vi "DynamicLoadLRvi.vi"(0 "LibName\\viName":string="CRC与诊断.lvlibp\\CRC与诊断\\CRC类\\CRC计算.vi", 1 "校验算法名称":string="Anti_Add", 2 "校验数据":u8[](array[numeric])=[215, 130, 0, 0, 0, 0, 11, 0] format="%x", 3 "校验长度":u8=7) -> (14 "校验值":u64=7)   [LabVIEW 2020]
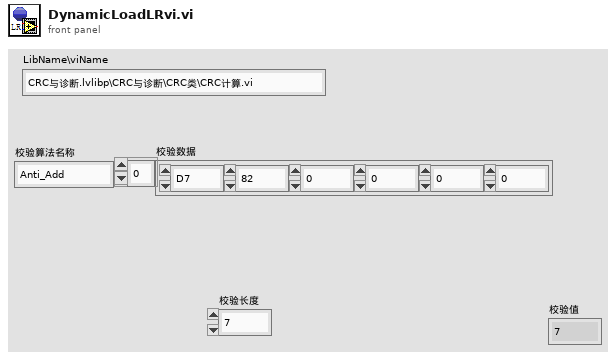
[diagram p1: front panel]
types:
  T1 = enum32{"invalid app kind", "Development System", "Run Time System", "Student Edition", "Embedded LabVIEW", "Evaluation", "Custom"}
  T2 = enum32{"Invalid", "Standard", "Closed", "Hidden", "Minimized", "Maximized"}
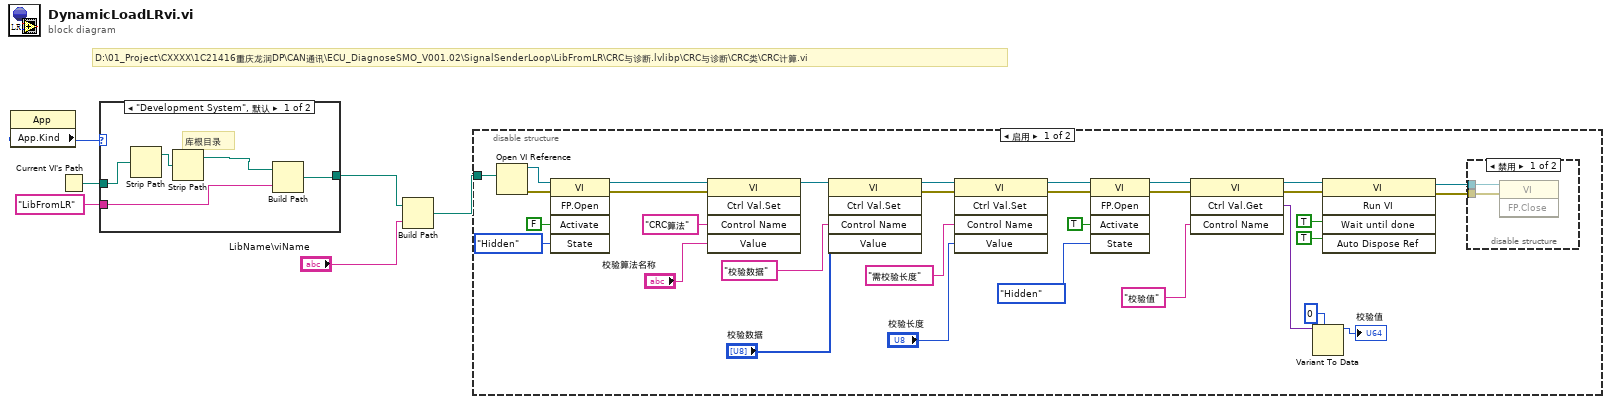
[diagram p0: block diagram]
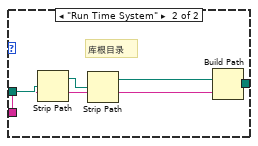
[diagram p4: hidden frame]
diagram:
  # "D:\\01_Project\\CXXXX\\1C21416重庆龙润DP\\CAN通讯\\ECU_DiagnoseSMO_V001.02\\SignalSenderLoop\\LibFromLR\\CRC与诊断.lvlibp\\CRC与诊断\\CRC类\\CRC计算.vi"
  n1 = property class="App"() -> ("App.Kind"=w4:T1)  [unwired: 2 in, 2 out]
  n2 = Current VI's Path() -> (path=w5:path)
  n3 = case shown="\"Development System\", 默认" w4 {
    tunnel: w5 -> [w11 w16]
    tunnel: [w8 w12] -> w3
    tunnel: "LibFromLR" ("ConfigFlieFolderName") -> [w7 w13]
    frame "Development System", Default {
      # "库根目录"
      n4 = Strip Path(path=w11) -> (stripped path=w10:path)  [unwired: 1 out]
      n5 = Strip Path(path=w10) -> (stripped path=w9:path)  [unwired: 1 out]
      n6 = Build Path(base path=w9, name or relative path=w7) -> (appended path=w8:path)
    }
    frame "Run Time System" {
      # "库根目录"
      n7 = Strip Path(path=w16) -> (stripped path=w15:path)  [unwired: 1 out]
      n8 = Strip Path(path=w15) -> (stripped path=w14:path)  [unwired: 1 out]
      n9 = Build Path(base path=w14, name or relative path=w13) -> (appended path=w12:path)
    }
  }
  n10 = Build Path(base path=w3, name or relative path="LibName\\viName") -> (appended path=w1:path)
  n11 = disable-structure shown="启用" {
    disable-tunnel: w1 -> [w36 _]
    frame Enabled {
      n12 = Open VI Reference(vi path=w36) -> (vi reference=w47:refnum<vi>, error out=w48:errorcluster)  [unwired: 5 in]
      n13 = invoke class="VI" method="FP.Open"(reference=w47, error in=w48, "Activate"=FALSE ("激活？"), "State"=T2."Hidden" ("状态")) -> (reference out=w43:refnum<vi>, error out=w46:errorcluster)  [unwired: 1 in, 3 out]
      n14 = invoke class="VI" method="Ctrl Val.Set"(reference=w43, error in=w46, "Control Name"="CRC算法" ("控件名"), "Value"="校验算法名称") -> (reference out=w34:refnum<vi>)  [unwired: 1 in, 4 out]
      n15 = invoke class="VI" method="Ctrl Val.Set"(reference=w34, "Control Name"="校验数据" ("控件名"), "Value"="校验数据") -> (reference out=w33:refnum<vi>, error out=w32:errorcluster)  [unwired: 2 in, 3 out]
      n16 = invoke class="VI" method="Ctrl Val.Set"(reference=w33, error in=w32, "Control Name"="需校验长度" ("控件名"), "Value"="校验长度") -> (reference out=w29:refnum<vi>, error out=w28:errorcluster)  [unwired: 1 in, 3 out]
      n17 = invoke class="VI" method="FP.Open"(reference=w29, error in=w28, "Activate"=TRUE ("激活？"), "State"=T2."Hidden" ("状态")) -> (reference out=w42:refnum<vi>, error out=w41:errorcluster)  [unwired: 1 in, 3 out]
      n18 = invoke class="VI" method="Ctrl Val.Get"(reference=w42, error in=w41, "Control Name"="校验值" ("控件名")) -> (reference out=w40:refnum<vi>, error out=w39:errorcluster, "Get Control Value Variant"=w22:variant)  [unwired: 1 in, 1 out]
      n19 = Variant To Data(type=u64 0 ("校验值"), Variant=w22) -> (data=→"校验值":u64)  [unwired: 1 in, 1 out]
      n20 = invoke class="VI" method="Run VI"(reference=w40, error in=w39, "Wait until done"=TRUE ("Wait Until Done"), "Auto Dispose Ref"=TRUE ("Auto Dispose Reference")) -> (reference out=w18:refnum<vi>, error out=w17:errorcluster)  [unwired: 1 in, 3 out]
      n21 = disable-structure shown="禁用" {
        disable-tunnel: w18 -> [w50 _]
        disable-tunnel: w17 -> [w49 _]
        frame Disabled {
          n22 = invoke class="VI" method="FP.Close"(reference=w50, error in=w49) -> ()  [unwired: 1 in, 3 out]
        }
        frame Enabled {
        }
      }
    }
    frame Disabled {
    }
  }
